vi "browse.vi"(8 "stop":bool, 9 "index (page)":i32(slide)=200 scale=0.0..512.0, 10 "Array":i32[][][](array[numeric])) -> (1 "Waveform Graph":u16[](graph), 2 "Intensity Graph":u16[][](graph))   [LabVIEW 2016]
panel:
  in  "file path (use dialog)":path=path "D:/All users/PoSheng/acuisition0727/LEDonColorPatternBinary.txt"
  out "max value":u16
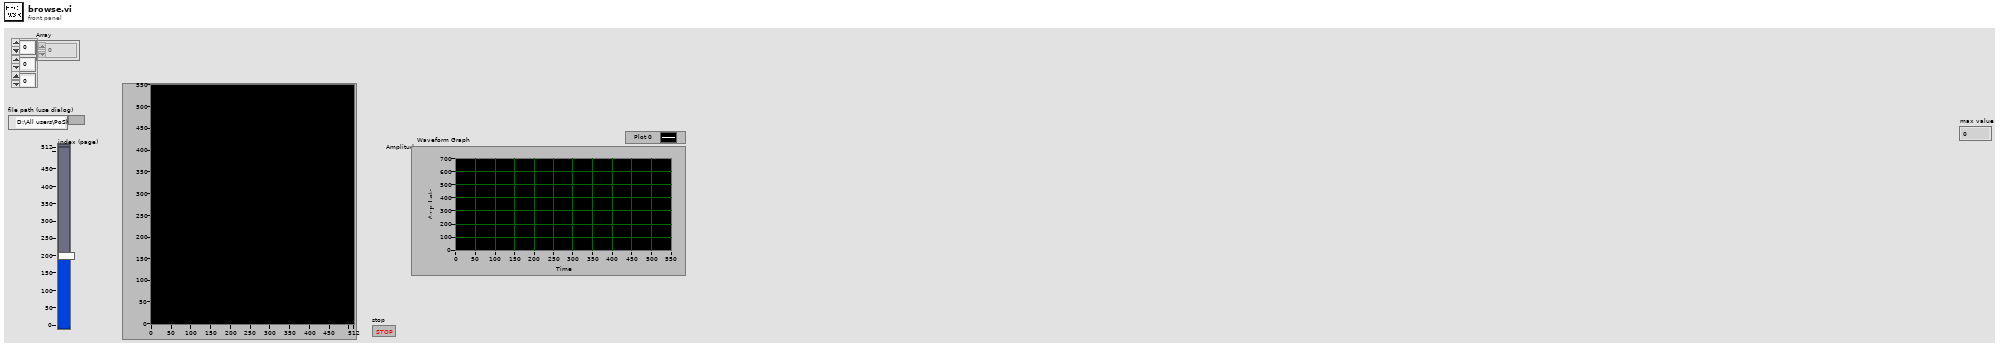
[diagram p1: front panel]
types:
  T1 = enum16{"big-endian, network order", "native, host order", "little-endian"}
  T2 = typedef "LVPoint32TypeDef.ctl" = cluster{"Horizontal":i32, "Vertical":i32}
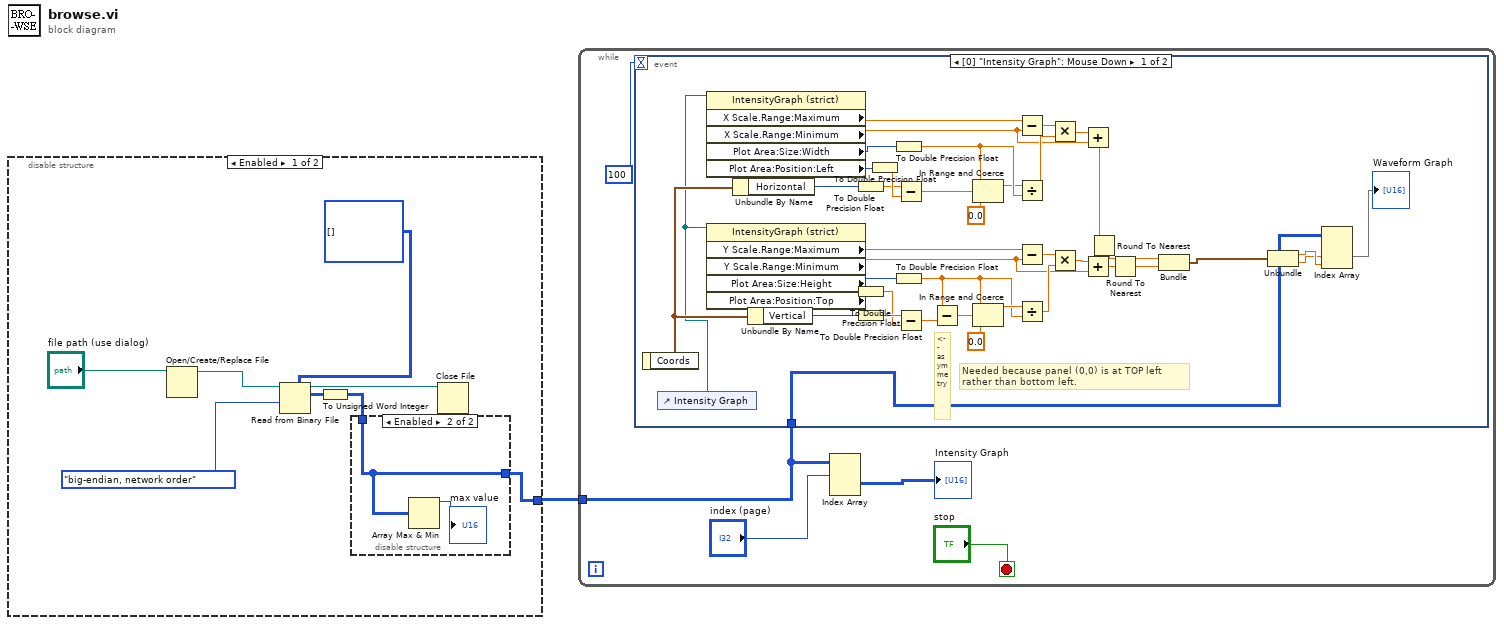
[diagram p0: block diagram]
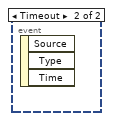
[diagram p2: hidden frame]
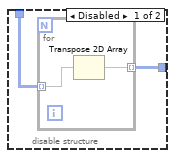
[diagram p3: hidden frame]
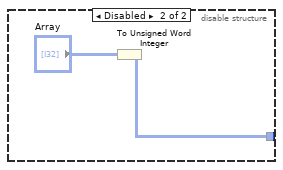
[diagram p4: hidden frame]
diagram:
  n1 = disable-structure shown="Enabled" {
    disable-tunnel: [w2 w16] -> w1
    frame Enabled {
      n2 = Open/Create/Replace File(file path (use dialog)="file path (use dialog)") -> (refnum out=w8:refnum<file>)  [unwired: 5 in, 2 out]
      n3 = Read from Binary File(5:i32[][][] [], 9:T1."big-endian, network order" ("byte order (0:big-endian, network order)"), 11:w8) -> (2:w4:i32[][][], 3:w7:refnum<file>)  [unwired: 3 in, 2 out]
      n4 = To Unsigned Word Integer(number=w4) -> (unsigned 16bit integer=w3:u16[][][])
      n5 = disable-structure shown="Enabled" {
        disable-tunnel: w3 -> [w11 w15]
        disable-tunnel: [w10 w15] -> w2
        frame Disabled {
          n6 = for {
            tunnel: w11 -> [w13] mode=indexing
            tunnel: [w12] -> w10 mode=indexing
            n7 = Transpose 2D Array(2D array=w13) -> (transposed array=w12:u16[][])
          }
        }
        frame Enabled {
          n8 = Array Max & Min(array=w15) -> (max value=→"max value":u16)  [unwired: 3 out]
        }
      }
      n9 = Close File(refnum=w7) -> ()  [unwired: 1 in, 2 out]
    }
    frame Disabled {
      n10 = To Unsigned Word Integer(number="Array") -> (unsigned 16bit integer=w16:u16[][][])
    }
  }
  n11 = while {
    tunnel: w1 -> [w19]
    stop <- "stop" stop-if-true
    n12 = event shown="[0] \"Intensity Graph\": Mouse Down" {
      selector: _ -> [_ _]
      dyn-events: _ -> [_ _]
      timeout: 100 -> [_ _]
      tunnel: w19 -> [w62 _]
      event "Intensity Graph": Mouse Down {
        # "<-- asymmetry"
        # "Needed because panel (0,0) is at TOP left rather than bottom left."
        n13 = event-data() -> ("Coords"=w29:T2)  [unwired: 1 in]
        n14 = control-ref of="Intensity Graph"() -> (w28:refnum<vi>)
        n15 = property on="Property Node" class="IntensityGraph (strict)"(reference=w28) -> ("X Scale.Range:Maximum"=w36:dbl, "X Scale.Range:Minimum"=w35:dbl, "Plot Area:Size:Width"=w34:u32, "Plot Area:Position:Left"=w33:i32)  [unwired: 1 in, 2 out]
        n16 = property on="Property Node" class="IntensityGraph (strict)"(reference=w28) -> ("Y Scale.Range:Maximum"=w60:dbl, "Y Scale.Range:Minimum"=w55:dbl, "Plot Area:Size:Height"=w52:u32, "Plot Area:Position:Top"=w45:i32)  [unwired: 1 in, 2 out]
        n17 = Unbundle By Name(w29) -> ("Horizontal"=w32:i32)
        n18 = Unbundle By Name(w29) -> ("Vertical"=w59:i32)
        n19 = To Double Precision Float(number=w32) -> (double precision float=w40:dbl)
        n20 = To Double Precision Float(number=w45) -> (double precision float=w50:dbl)
        n21 = To Double Precision Float(number=w59) -> (double precision float=w51:dbl)
        n22 = To Double Precision Float(number=w33) -> (double precision float=w41:dbl)
        n23 = To Double Precision Float(number=w34) -> (double precision float=w44:dbl)
        n24 = To Double Precision Float(number=w52) -> (double precision float=w46:dbl)
        n25 = Subtract(x=w40, y=w41) -> (x-y=w30:dbl)
        n26 = Subtract(x=w51, y=w50) -> (x-y=w53:dbl)
        n27 = Subtract(x=w46, y=w53) -> (x-y=w49:dbl)
        n28 = In Range and Coerce(upper limit=w44, x=w30, lower limit=0.0) -> (coerced(x)=w43:dbl)  [unwired: 1 out]
        n29 = In Range and Coerce(upper limit=w46, x=w49, lower limit=0.0) -> (coerced(x)=w47:dbl)  [unwired: 1 out]
        n30 = Subtract(x=w36, y=w35) -> (x-y=w37:dbl)
        n31 = Divide(x=w43, y=w44) -> (x/y=w38:dbl)
        n32 = Subtract(x=w60, y=w55) -> (x-y=w58:dbl)
        n33 = Divide(x=w47, y=w46) -> (x/y=w57:dbl)
        n34 = Multiply(x=w37, y=w38) -> (x*y=w39:dbl)
        n35 = Multiply(x=w58, y=w57) -> (x*y=w56:dbl)
        n36 = Add(x=w39, y=w35) -> (x+y=w31:dbl)
        n37 = Add(x=w56, y=w55) -> (x+y=w54:dbl)
        n38 = Round To Nearest(number=w31) -> (nearest integer value=w23:dbl)
        n39 = Round To Nearest(number=w54) -> (nearest integer value=w24:dbl)
        n40 = Bundle(w23, w24) -> (w27:cluster{dbl, dbl})  [unwired: 1 in]
        n41 = Unbundle(w27) -> (w26:dbl, w25:dbl)
        n42 = Index Array(array=w62, index (dim 1)=w25, index (dim 2)=w26) -> (element=→"Waveform Graph":u16[])  [unwired: 1 in]
      }
      event Timeout {
        n43 = event-data() -> ()  [unwired: 1 in, 3 out]
      }
    }
    n44 = Index Array(array=w19, index (dim 0)="index (page)") -> (element=→"Intensity Graph":u16[][])  [unwired: 2 in]
  }
